vi "Untitledpass.vi"(0 "vi path":path) -> (4 "vi path 2":path, 15 "true":bool)   [LabVIEW 2015]
panel:
  out "Skip":bool
  out "Contents":string[][](array[string])
  in  "Cancel":bool
  in  "OK Button":bool
  in  "Password":string
  in  "User Name":string
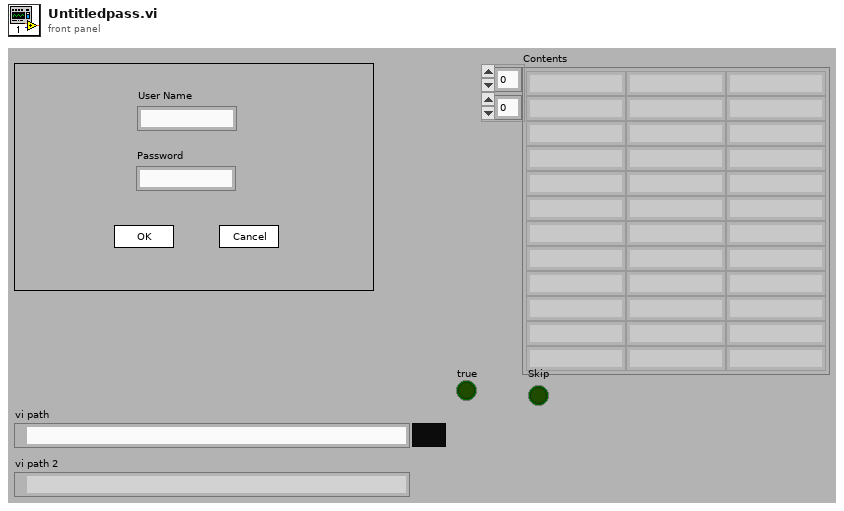
[diagram p1: front panel]
types:
  T1 = enum16{"open", "open or create", "create or replace", "create", "open (read only)"}
  T2 = enum16{"Left Button", "Center Button", "Right Button", "Window Close"}
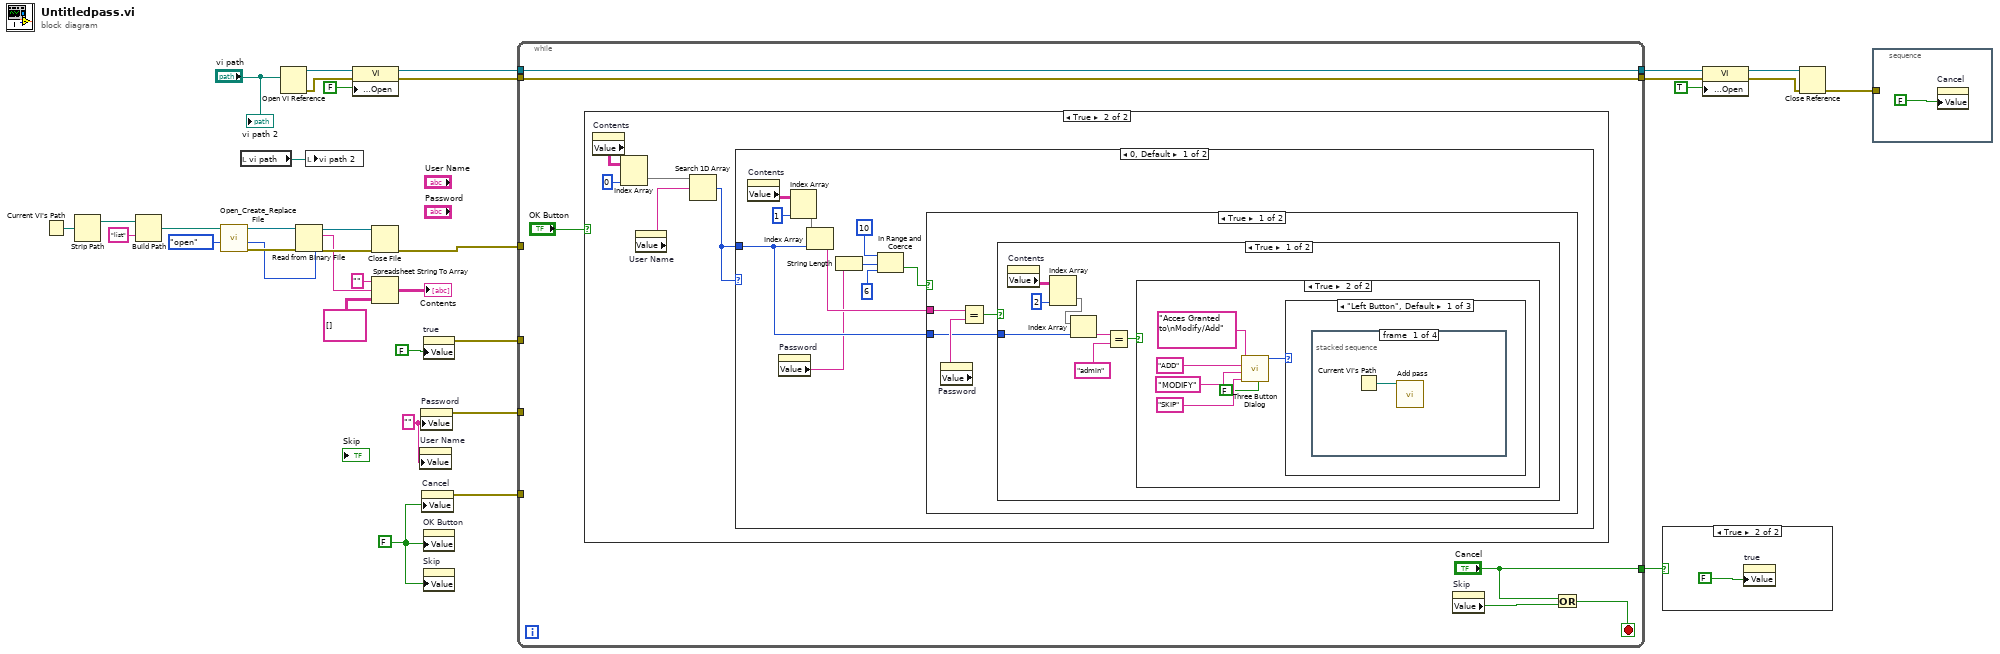
[diagram p0: block diagram]
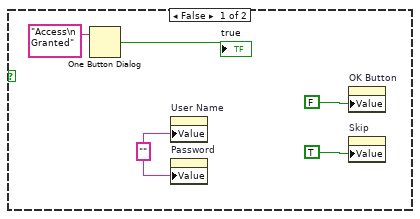
[diagram p4: hidden frame]
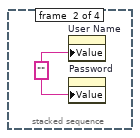
[diagram p5: hidden frame]
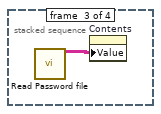
[diagram p6: hidden frame]
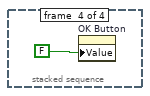
[diagram p7: hidden frame]
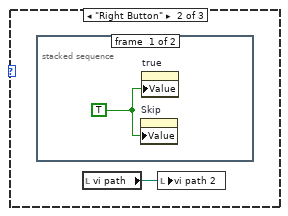
[diagram p8: hidden frame]
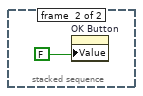
[diagram p9: hidden frame]
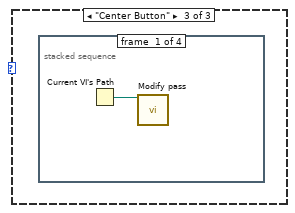
[diagram p10: hidden frame]
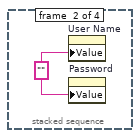
[diagram p11: hidden frame]
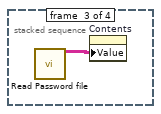
[diagram p12: hidden frame]
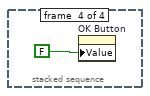
[diagram p13: hidden frame]
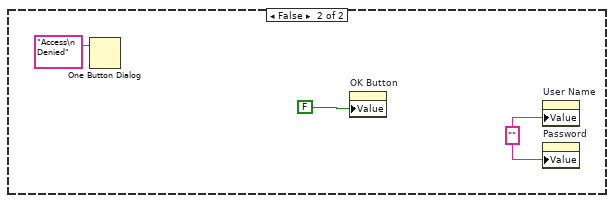
[diagram p14: hidden frame]
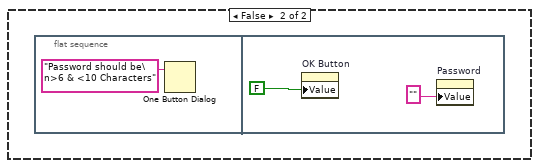
[diagram p15: hidden frame]
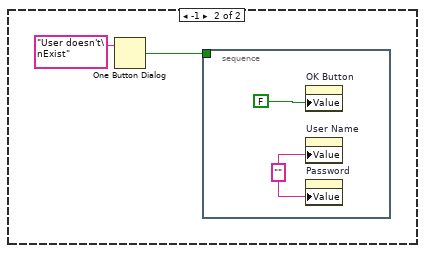
[diagram p16: hidden frame]
diagram:
  w6 = FALSE ("true")
  w35 = "" ("Password")
  n1 = Current VI's Path() -> (path=w4:path)
  n2 = Strip Path(path=w4) -> (stripped path=w3:path)  [unwired: 1 out]
  n3 = Build Path(base path=w3, name or relative path="list") -> (appended path=w1:path)
  n4 = call <vilib>:"Open_Create_Replace File.vi"("function (open:0)"=T1."open", "file path"=w1) -> ("error out"=w33:errorcluster, "file size (bytes)"=w29:i32, "refnum"=w32:refnum<file>)  [unwired: 6 in, 1 out]
  n5 = local read "vi path"() -> (w10:path)
  n6 = Open VI Reference(vi path="vi path") -> (vi reference=w20:refnum<vi>, error out=w19:errorcluster)  [unwired: 5 in]
  n7 = Read from Binary File(8:w33, 10:w29, 11:w32) -> (0:w31:errorcluster, 2:w28:string, 3:w30:refnum<file>)  [unwired: 3 in, 1 out]
  n8 = local write "vi path 2"(w10) -> ()
  n9 = property class="VI"(reference=w20, error in=w19, "Front Panel Window:Open"=FALSE) -> (reference out=w17:refnum<vi>, error out=w16:errorcluster)
  n10 = Close File(refnum=w30, error in=w31) -> (error out=w26:errorcluster)  [unwired: 1 out]
  n11 = Spreadsheet String To Array(format string="", spreadsheet string=w28, array type (2D Dbl)=string[][] []) -> (array=→"Contents":string[][])  [unwired: 1 in]
  n12 = property on="User Name" class="Str"("Value"=w35) -> ()  [unwired: 2 in, 2 out]
  n13 = property on="Password" class="Str"("Value"=w35) -> (error out=w34:errorcluster)  [unwired: 2 in, 1 out]
  n14 = property on="Cancel" class="Bool (strict)"("Value"=w6) -> (error out=w9:errorcluster)  [unwired: 2 in, 1 out]
  n15 = property on="true" class="Bool (strict)"("Value"=FALSE ("true")) -> (error out=w22:errorcluster)  [unwired: 2 in, 1 out]
  n16 = property on="OK Button" class="Bool (strict)"("Value"=w6) -> ()  [unwired: 2 in, 2 out]
  n17 = property on="Skip" class="Bool (strict)"("Value"=w6) -> ()  [unwired: 2 in, 2 out]
  n18 = while {
    tunnel: w34 -> [_]
    tunnel: w26 -> [_]
    tunnel: w22 -> [_]
    tunnel: w17 -> [w40]
    tunnel: w16 -> [w39]
    tunnel: [w40] -> w14
    tunnel: [w39] -> w13
    tunnel: w9 -> [_]
    tunnel: ["Cancel"] -> w7
    stop <- w36 stop-if-true
    n19 = case shown="True" "OK Button" {
      frame False {
      }
      frame True {
        n20 = property on="Contents" class="Arr (strict)"() -> ("Value"=w44:string[][])  [unwired: 2 in, 2 out]
        n21 = Index Array(array=w44, index (col)=0 ("disabled index (col)")) -> (element=w42:string[])  [unwired: 1 in]
        n22 = property on="User Name" class="Str"() -> ("Value"=w46:string)  [unwired: 2 in, 2 out]
        n23 = Search 1D Array(1D array=w42, element=w46) -> (index of element=w45:i32)  [unwired: 1 in]
        n24 = case shown="0, Default" w45 {
          tunnel: w45 -> [w51 _]
          frame 0, Default {
            n25 = property on="Contents" class="Arr (strict)"() -> ("Value"=w49:string[][])  [unwired: 2 in, 2 out]
            n26 = property on="Password" class="Str"() -> ("Value"=w47:string)  [unwired: 2 in, 2 out]
            n27 = Index Array(array=w49, index (col)=1 ("disabled index (col)")) -> (element=w48:string[])  [unwired: 1 in]
            n28 = Index Array(array=w48, index=w51) -> (element=w52:string)
            n29 = String Length(string=w47) -> (length=w56:i32)
            n30 = In Range and Coerce(upper limit=10, x=w56, lower limit=6) -> (In Range?=w53:bool)  [unwired: 1 out]
            n31 = case shown="True" w53 {
              tunnel: w52 -> [w59 _]
              tunnel: w51 -> [w57 _]
              frame True {
                n32 = property on="Password" class="Str"() -> ("Value"=w60:string)  [unwired: 2 in, 2 out]
                n33 = Equal?(x=w59, y=w60) -> (x = y?=w58:bool)
                n34 = case shown="True" w58 {
                  tunnel: w57 -> [w67 _]
                  frame True {
                    n35 = property on="Contents" class="Arr (strict)"() -> ("Value"=w63:string[][])  [unwired: 2 in, 2 out]
                    n36 = Index Array(array=w63, index (col)=2 ("disabled index (col)")) -> (element=w61:string[])  [unwired: 1 in]
                    n37 = Index Array(array=w61, index=w67) -> (element=w66:string)
                    n38 = Equal?(x=w66, y="admin") -> (x = y?=w64:bool)
                    n39 = case shown="True" w64 {
                      frame False {
                        w71 = "" ("Password")
                        n40 = One Button Dialog(message="Access\n Granted") -> (true=→"true":bool)  [unwired: 1 in]
                        n41 = property on="User Name" class="Str"("Value"=w71) -> ()  [unwired: 2 in, 2 out]
                        n42 = property on="Password" class="Str"("Value"=w71) -> ()  [unwired: 2 in, 2 out]
                        n43 = property on="OK Button" class="Bool (strict)"("Value"=FALSE ("true")) -> ()  [unwired: 2 in, 2 out]
                        n44 = property on="Skip" class="Bool (strict)"("Value"=TRUE ("Skip")) -> ()  [unwired: 2 in, 2 out]
                      }
                      frame True {
                        n45 = call <vilib>:"Three Button Dialog.vi"("Allow user to close window? (TRUE)"=FALSE, "Right Button Text (\"Cancel\")"="SKIP" ("Left Button Text (\"Yes\")"), "Center Button Text (\"No\")"="MODIFY" ("Left Button Text (\"Yes\")"), "Left Button Text (\"Yes\")"="ADD" ("Left Button Text (\"Yes\")"), "message"="Acces Granted to\nModify/Add") -> ("Which Button?"=w75:T2)  [unwired: 6 in]
                        n46 = case shown="\"Left Button\", Default" w75 {
                          frame "Left Button", Default {
                            n47 = stacked-sequence {
                              frame #0 {
                                n48 = Current VI's Path() -> (path=w79:path)
                                n49 = call "Add pass.vi"("vi path"=w79) -> ()  [unwired: 15 in]
                              }
                              frame #1 {
                                w80 = "" ("Password")
                                n50 = property on="User Name" class="Str"("Value"=w80) -> ()  [unwired: 2 in, 2 out]
                                n51 = property on="Password" class="Str"("Value"=w80) -> ()  [unwired: 2 in, 2 out]
                              }
                              frame #2 {
                                n52 = call "Read Password file.vi"() -> ("Contents"=w81:string[][])  [unwired: 15 in]
                                n53 = property on="Contents" class="Arr (strict)"("Value"=w81) -> ()  [unwired: 2 in, 2 out]
                              }
                              frame #3 {
                                n54 = property on="OK Button" class="Bool (strict)"("Value"=FALSE ("true")) -> ()  [unwired: 2 in, 2 out]
                              }
                            }
                          }
                          frame "Right Button" {
                            n55 = stacked-sequence {
                              frame #0 {
                                w84 = TRUE ("true")
                                n56 = property on="Skip" class="Bool (strict)"("Value"=w84) -> ()  [unwired: 2 in, 2 out]
                                n57 = property on="true" class="Bool (strict)"("Value"=w84) -> ()  [unwired: 2 in, 2 out]
                              }
                              frame #1 {
                                n58 = property on="OK Button" class="Bool (strict)"("Value"=FALSE ("true")) -> ()  [unwired: 2 in, 2 out]
                              }
                            }
                            n59 = local read "vi path"() -> (w83:path)
                            n60 = local write "vi path 2"(w83) -> ()
                          }
                          frame "Center Button" {
                            n61 = stacked-sequence {
                              frame #0 {
                                n62 = Current VI's Path() -> (path=w86:path)
                                n63 = call "Modify pass.vi"("vi path"=w86) -> ()  [unwired: 15 in]
                              }
                              frame #1 {
                                w87 = "" ("Password")
                                n64 = property on="User Name" class="Str"("Value"=w87) -> ()  [unwired: 2 in, 2 out]
                                n65 = property on="Password" class="Str"("Value"=w87) -> ()  [unwired: 2 in, 2 out]
                              }
                              frame #2 {
                                n66 = call "Read Password file.vi"() -> ("Contents"=w88:string[][])  [unwired: 15 in]
                                n67 = property on="Contents" class="Arr (strict)"("Value"=w88) -> ()  [unwired: 2 in, 2 out]
                              }
                              frame #3 {
                                n68 = property on="OK Button" class="Bool (strict)"("Value"=FALSE ("true")) -> ()  [unwired: 2 in, 2 out]
                              }
                            }
                          }
                        }
                      }
                    }
                  }
                  frame False {
                    w91 = "" ("Password")
                    n69 = One Button Dialog(message="Access\n Denied") -> ()  [unwired: 1 in, 1 out]
                    n70 = property on="OK Button" class="Bool (strict)"("Value"=FALSE ("true")) -> ()  [unwired: 2 in, 2 out]
                    n71 = property on="User Name" class="Str"("Value"=w91) -> ()  [unwired: 2 in, 2 out]
                    n72 = property on="Password" class="Str"("Value"=w91) -> ()  [unwired: 2 in, 2 out]
                  }
                }
              }
              frame False {
                n73 = flat-sequence {
                  frame #0 {
                    n74 = One Button Dialog(message="Password should be\n>6 & <10 Characters") -> ()  [unwired: 1 in, 1 out]
                  }
                  frame #1 {
                    n75 = property on="OK Button" class="Bool (strict)"("Value"=FALSE ("true")) -> ()  [unwired: 2 in, 2 out]
                    n76 = property on="Password" class="Str"("Value"="" ("Password")) -> ()  [unwired: 2 in, 2 out]
                  }
                }
              }
            }
          }
          frame -1 {
            n77 = One Button Dialog(message="User doesn't\nExist") -> (true=w96:bool)  [unwired: 1 in]
            n78 = stacked-sequence {
              tunnel: w96 -> [_]
              frame #0 {
                w98 = "" ("Password")
                n79 = property on="OK Button" class="Bool (strict)"("Value"=FALSE ("true")) -> ()  [unwired: 2 in, 2 out]
                n80 = property on="User Name" class="Str"("Value"=w98) -> ()  [unwired: 2 in, 2 out]
                n81 = property on="Password" class="Str"("Value"=w98) -> ()  [unwired: 2 in, 2 out]
              }
            }
          }
        }
      }
    }
    n82 = property on="Skip" class="Bool (strict)"() -> ("Value"=w37:bool)  [unwired: 2 in, 2 out]
    n83 = Or(x="Cancel", y=w37) -> (x .or. y?=w36:bool)
  }
  n84 = case shown="True" w7 {
    frame False {
    }
    frame True {
      n85 = property on="true" class="Bool (strict)"("Value"=FALSE ("true")) -> ()  [unwired: 2 in, 2 out]
    }
  }
  n86 = property class="VI"(reference=w14, error in=w13, "Front Panel Window:Open"=TRUE) -> (reference out=w12:refnum<vi>, error out=w11:errorcluster)
  n87 = Close Reference(reference=w12, error in (no error)=w11) -> (error out=w8:errorcluster)
  n88 = stacked-sequence {
    tunnel: w8 -> [_]
    frame #0 {
      n89 = property on="Cancel" class="Bool (strict)"("Value"=FALSE ("true")) -> ()  [unwired: 2 in, 2 out]
    }
  }
  "vi path 2" <- "vi path"
